vi "Read Subscribe Msg.vi"(11 "IObserver in":refnum<class "IObserver.lvclass">) -> (2 "Pre-Addressed Subscribe Msg":refnum<class "Subscribe Msg.lvclass">)   [LabVIEW 2017, in "IObserver.lvlib" / "IObserver.lvclass"]
uses:
  IObserver.lvclass
  IMediator/IMediator Messages/Subscribe Msg/Subscribe Msg.lvclass
  IObserver.lvclass/IObserver.ctl
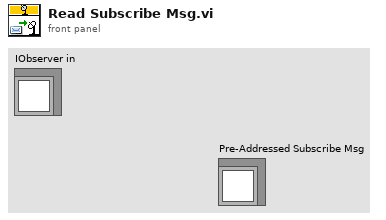
[diagram p1: front panel]
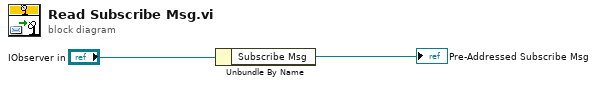
[diagram p0: block diagram]
diagram:
  n1 = Unbundle By Name("IObserver in") -> ("Subscribe Msg"=→"Pre-Addressed Subscribe Msg":refnum<class "Subscribe Msg.lvclass">)
